vi "PIDTEMPtest2.vi"() -> ()   [LabVIEW 2015]
uses:
  <vilib>/DAQmx/read.llb/DAQmx Read (Analog 1D Wfm NChan 1Samp).vi
  <vilib>/Analysis/baseanly.llb/Mean (DBL).vi
  <vilib>/DAQmx/write.llb/DAQmx Write (Digital 1D Bool NChan 1Samp 1Line).vi
  <vilib>/DAQmx/miscellaneous.llb/DAQmx Fill In Error Info.vi
  <vilib>/addons/control/pid/pid.llb/PID Advanced (DBL).vi
  <vilib>/addons/control/pid/NI_PID_pid.lvlib
  <vilib>/Analysis/NI_AALBase.lvlib
panel:
  out "Temp":dbl
  out "Numeric":i32
  out "Duty Cycle %":dbl
  in  "reinitialize? (F)":bool
  out "Voltage Reading(Temp)":dbl format="%#_13g"
  out "Temperature (Celcius)":dbl format="%#.1g"
  out "Temp(C)":dbl(slide) scale=-10.0..100.0
  out "Temp Chart":waveform(dbl)(graph)
  out "Temp Chart 2":waveform(dbl)(graph)
  in  "Temp Setting":dbl
  in  "PID gains Temp":T1={"proportional gain (Kc)"=1.0, "integral time (Ti, min)"=0.01, "derivative time (Td, min)"=0.0} {"derivative time (Td, min)" format="%.3f"; "integral time (Ti, min)" format="%.3f"; "proportional gain (Kc)" format="%.3f"}
  in  "Stop Maintaining Temp":bool
  out "Control Value (Temp Sensor)":dbl(knob) scale=0.0..100.0
  in  "Steps in a cycle":i32=256
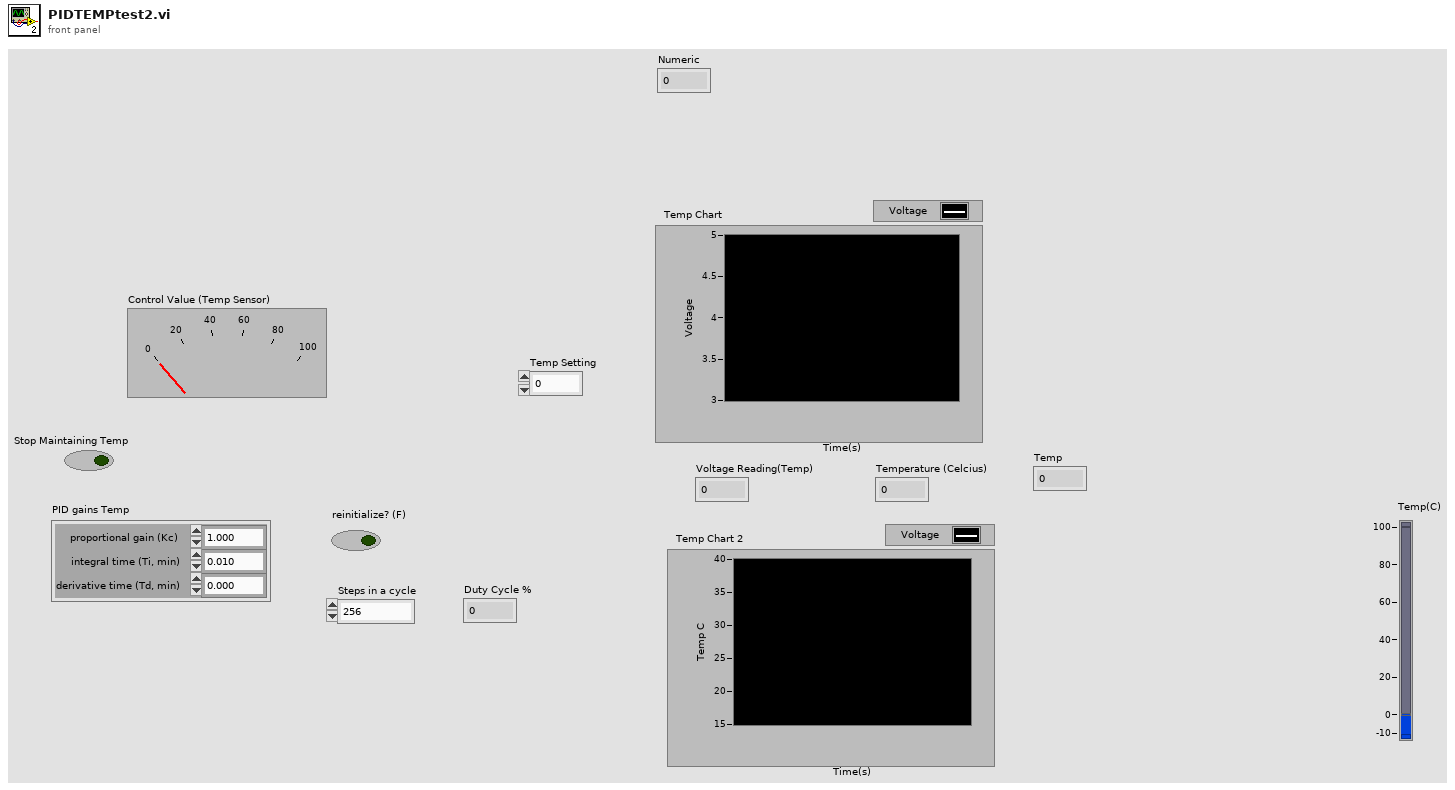
[diagram p1: front panel]
types:
  T1 = cluster{"proportional gain (Kc)":dbl, "integral time (Ti, min)":dbl, "derivative time (Td, min)":dbl}
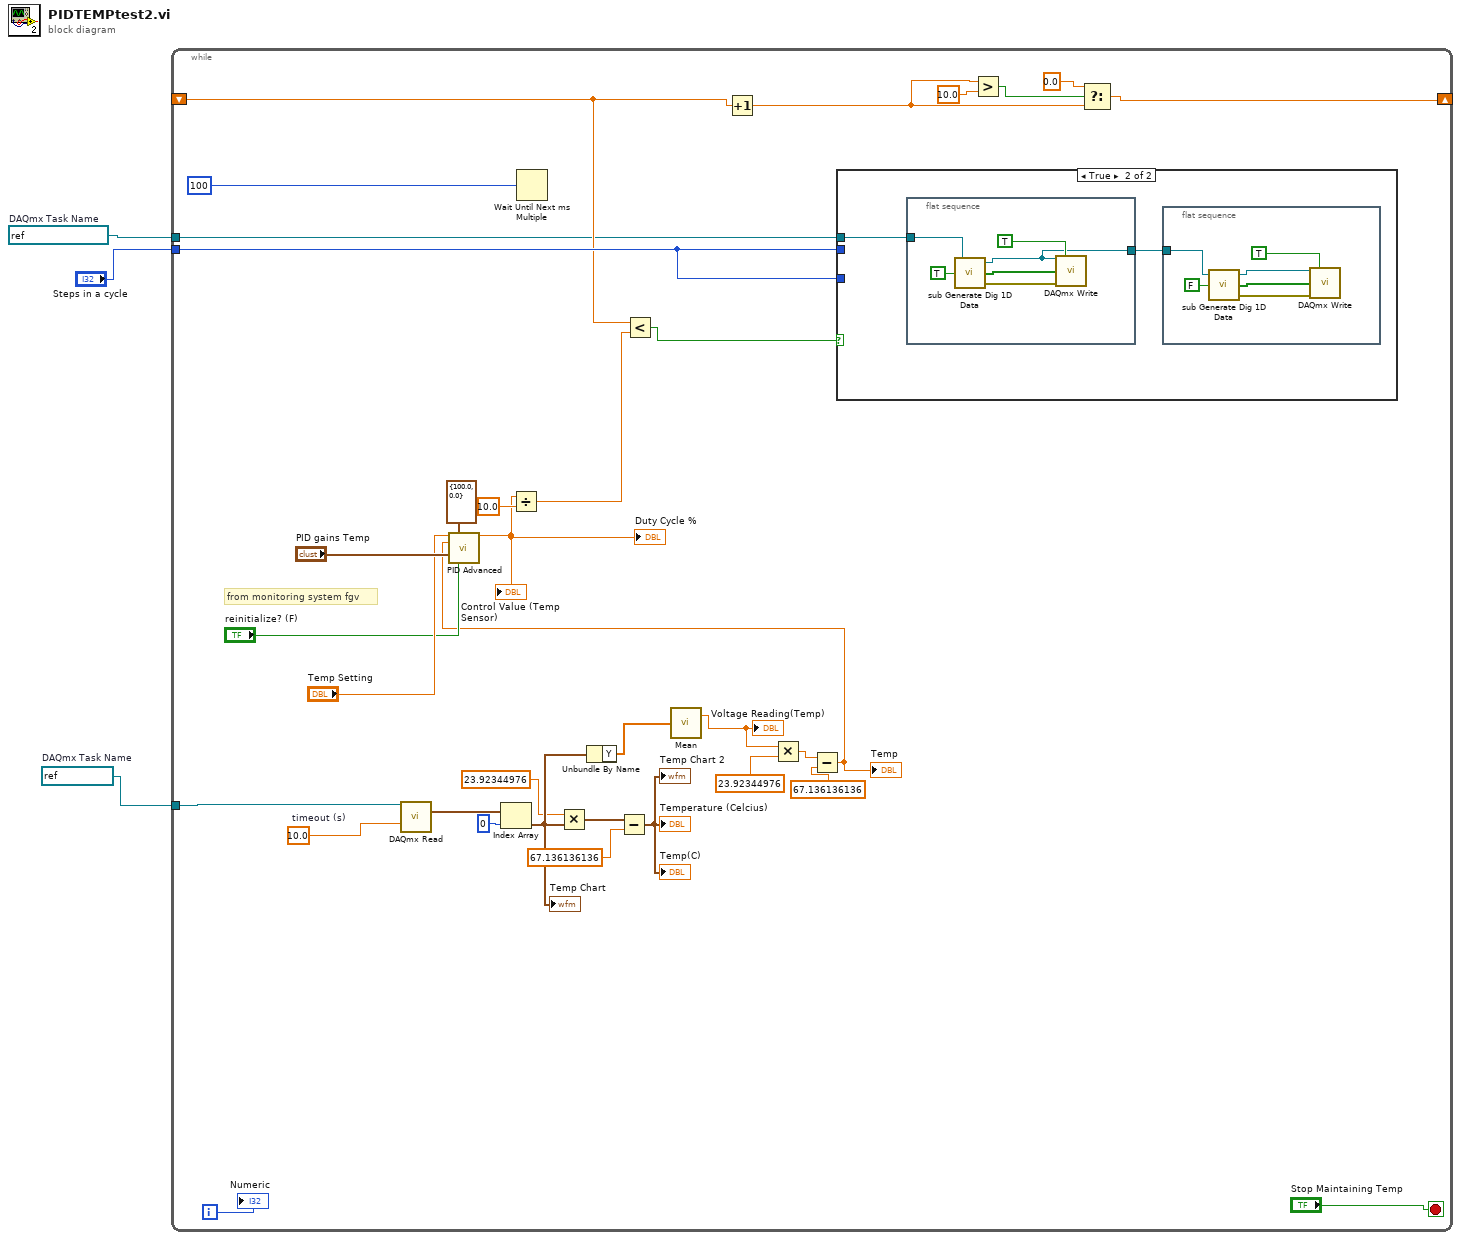
[diagram p0: block diagram]
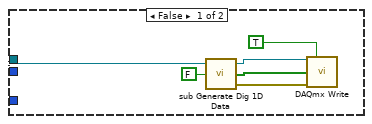
[diagram p2: hidden frame]
diagram:
  w1 = refnum<k21> "A0New1"  # DAQmx Task Name
  w3 = refnum<k21> "P0L0DigitalOut"  # DAQmx Task Name
  n1 = while {
    tunnel: w3 -> [w4]
    tunnel: "Steps in a cycle" -> [w36]
    tunnel: w1 -> [w17]
    shift-right: [w13] -> _
    shift-left: _ -> [w8]
    i -> [w31]
    stop <- "Stop Maintaining Temp" stop-if-true
    w18 = 10.0  # timeout (s)
    # "from monitoring system fgv"
    n2 = call-poly <vilib>:"DAQmx Read.vi"("task/channels in"=w17, "timeout"=w18) -> ("data"=w23:waveform(dbl)[])  [unwired: 11 in, 2 out]
    n3 = Index Array(array=w23, index=0) -> (element=w25:waveform(dbl))
    "Temp Chart" <- w25
    n4 = Wait Until Next ms Multiple(millisecond multiple=u32 100) -> ()  [unwired: 1 out]
    n5 = Multiply(x=23.92344976, y=w25) -> (x*y=w20:waveform(dbl))
    n6 = Unbundle By Name(w25) -> ("Y"=w26:dbl[])
    n7 = Subtract(x=w20, y=67.136136136) -> (x-y=→"Temperature (Celcius)" →"Temp(C)" →"Temp Chart 2":waveform(dbl))
    n8 = call-poly <vilib>:"Mean.vi"("X"=w26) -> ("mean"=w27:dbl)  [unwired: 1 out]
    "Voltage Reading(Temp)" <- w27
    n9 = Increment(x=w8) -> (x+1=w9:dbl)
    n10 = Multiply(x=w27, y=23.92344976) -> (x*y=w28:dbl)
    n11 = Subtract(x=w28, y=67.136136136) -> (x-y=w16:dbl)
    "Temp" <- w16
    n12 = call-poly <vilib>:"PID Advanced.vi"("setpoint"="Temp Setting", "output range"=cluster{"output high":dbl, "output low":dbl} {"output high"=100.0, "output low"=0.0}, "process variable"=w16, "PID gains"="PID gains Temp", "reinitialize? (F)"="reinitialize? (F)") -> ("output"=w5:dbl)  [unwired: 9 in, 1 out]
    "Control Value (Temp Sensor)" <- w5
    "Duty Cycle %" <- w5
    n13 = Divide(x=w5, y=10.0) -> (x/y=w7:dbl)
    n14 = Less?(x=w8, y=w7) -> (x < y?=w6:bool)
    n15 = case shown="True" w6 {
      tunnel: w4 -> [w39 w45]
      tunnel: w36 -> [_ _]
      tunnel: w36 -> [_ _]
      frame False {
        n16 = call <vilib>:"sub Generate Dig 1D Data.vi"("initial value"=FALSE, "task in"=w39) -> ("error out"=w42:errorcluster, "Data"=w40:bool[], "task out"=w41:refnum<k21>)  [unwired: 1 in]
        n17 = call-poly <vilib>:"DAQmx Write.vi"("task/channels in"=w41, "auto start"=TRUE, "data"=w40, "error in"=w42) -> ()  [unwired: 9 in, 3 out]
      }
      frame True {
        n18 = flat-sequence {
          tunnel: w45 -> [w53]
          tunnel: [w52] -> w44
          frame #0 {
            n19 = call <vilib>:"sub Generate Dig 1D Data.vi"("initial value"=TRUE, "task in"=w53) -> ("error out"=w55:errorcluster, "Data"=w56:bool[], "task out"=w52:refnum<k21>)  [unwired: 1 in]
            n20 = call-poly <vilib>:"DAQmx Write.vi"("task/channels in"=w52, "auto start"=TRUE, "data"=w56, "error in"=w55) -> ()  [unwired: 9 in, 3 out]
          }
        }
        n21 = flat-sequence {
          tunnel: w44 -> [w46]
          frame #0 {
            n22 = call <vilib>:"sub Generate Dig 1D Data.vi"("initial value"=FALSE, "task in"=w46) -> ("error out"=w50:errorcluster, "Data"=w48:bool[], "task out"=w49:refnum<k21>)  [unwired: 1 in]
            n23 = call-poly <vilib>:"DAQmx Write.vi"("task/channels in"=w49, "auto start"=TRUE, "data"=w48, "error in"=w50) -> ()  [unwired: 9 in, 3 out]
          }
        }
      }
    }
    n24 = Greater?(x=w9, y=10.0 ("x")) -> (0:w11:bool)
    n25 = Select(t=0.0, s=w11, f=w9) -> (s? t:f=w13:dbl)
    "Numeric" <- w31
  }
